vi "Test 4 Compare Same Types Higher With Joker.vi"(8 "error in (no error)":errorcluster, 11 "Test Case In":refnum<class "Day 7 Test.lvclass">) -> (0 "error out":errorcluster, 3 "Test Case Out":refnum<class "Day 7 Test.lvclass">)   [LabVIEW 2020, in "Day 7 Test.lvclass"]
uses:
  Day 7 Test.lvclass
  C:/Program Files (x86)/National Instruments/LabVIEW 2020/vi.lib/Astemes/LUnit/Test Case.lvclass
  <vilib>/Astemes/LUnit/Test Case.lvclass/Test Case.ctl
  <vilib>/Astemes/LUnit/Append Pass Result.vi
  <vilib>/Astemes/LUnit/Append Fail Result.vi
  Hand with Joker/Hand with Joker.lvclass
  <vilib>/Astemes/LUnit/Test Case.lvclass
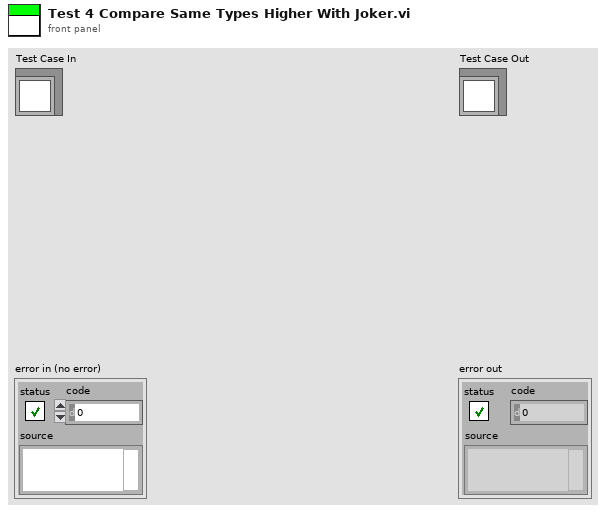
[diagram p1: front panel]
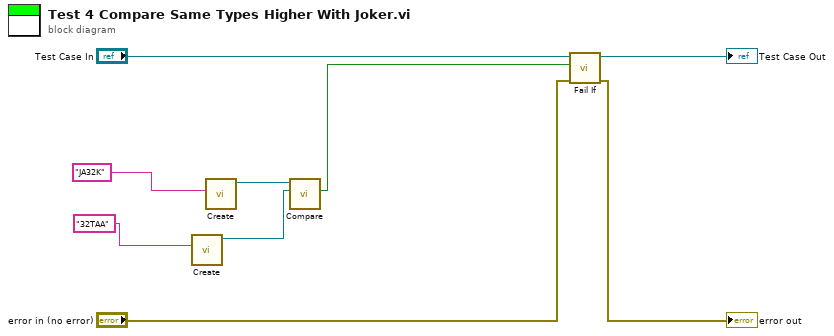
[diagram p0: block diagram]
diagram:
  n1 = call "Create.vi"("Input"="32TAA") -> ("Hand"=w4:refnum<class "Hand with Joker.lvclass">)  [unwired: 9 in, 1 out]
  n2 = call "Create.vi"("Input"="JA32K") -> ("Hand"=w5:refnum<class "Hand with Joker.lvclass">)  [unwired: 9 in, 1 out]
  n3 = call "Compare.vi"("Hand in 2"=w4, "Hand in"=w5) -> ("Higher?"=w3:bool)  [unwired: 7 in, 2 out]
  n4 = call <vilib>:"Fail If.vi"("error in (no error)"="error in (no error)", "Fail?"=w3, "LUnit Test Case In"="Test Case In") -> ("error out"=→"error out":errorcluster, "LUnit Test Case Out"=→"Test Case Out":refnum<class "Day 7 Test.lvclass">)  [unwired: 7 in]
